vi "DAC p PAA25 FP Conf.vi"(8 "error in (no error)":errorcluster, 9 "Used p PAA25":bool[](array[boolean]), 10 "Result Unit":string, 11 "DeepU Results in":refnum<class "DeepU Results.lvclass">) -> (0 "error out":errorcluster, 3 "DeepU Results out":refnum<class "DeepU Results.lvclass">)   [LabVIEW 2019, in "Results.lvlib" / "DeepU Results.lvclass"]
uses:
  DeepU Results.lvclass
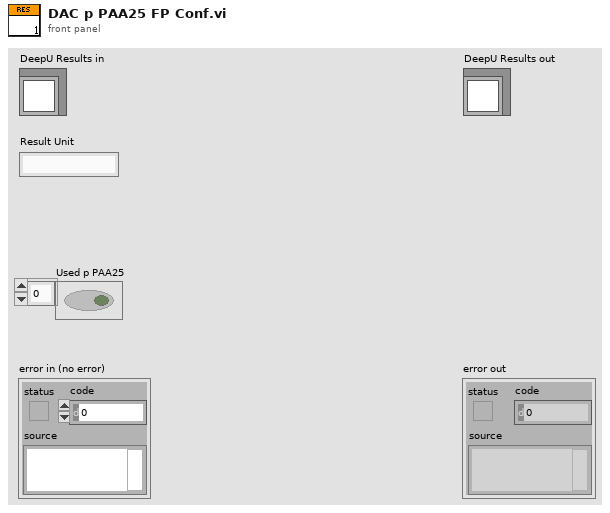
[diagram p1: front panel]
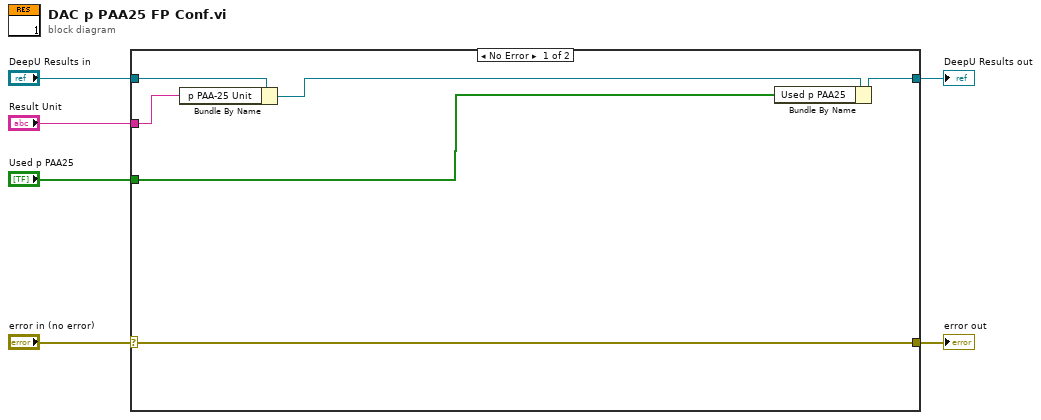
[diagram p0: block diagram]
diagram:
  n1 = case shown="No Error" "error in (no error)" {
    selector: "error in (no error)" -> [w12 w14]
    tunnel: [w12 w14] -> w5
    tunnel: [w8 w13] -> w3
    tunnel: "DeepU Results in" -> [w10 w13]
    tunnel: "Result Unit" -> [w9 _]
    tunnel: "Used p PAA25" -> [w7 _]
    frame No Error {
      n2 = Bundle By Name(cluster=w10, "p PAA-25 Unit"=w9) -> (w11:refnum<class "DeepU Results.lvclass">)
      n3 = Bundle By Name(cluster=w11, "Used p PAA25"=w7) -> (w8:refnum<class "DeepU Results.lvclass">)
    }
    frame Error {
    }
  }
  "error out" <- w5
  "DeepU Results out" <- w3
